vi "Check Device Type.vi"(8 "error in (no error)":errorcluster, 9 "Device Type Name":string, 10 "Device in":refnum<class "Device.lvclass">) -> (0 "error out":errorcluster, 1 "correct Device":bool, 2 "Device out":refnum<class "Device.lvclass">)   [LabVIEW 2011, in "Tinkerforge.lvlib" / "Device.lvclass"]
doc: "This VI is the parent class implementation of \"Check Device Type.vi\"."
uses:
  Device.lvclass
  IP Connection/Type Definitions/Errors.ctl
  IP Connection/IP Connection.lvclass
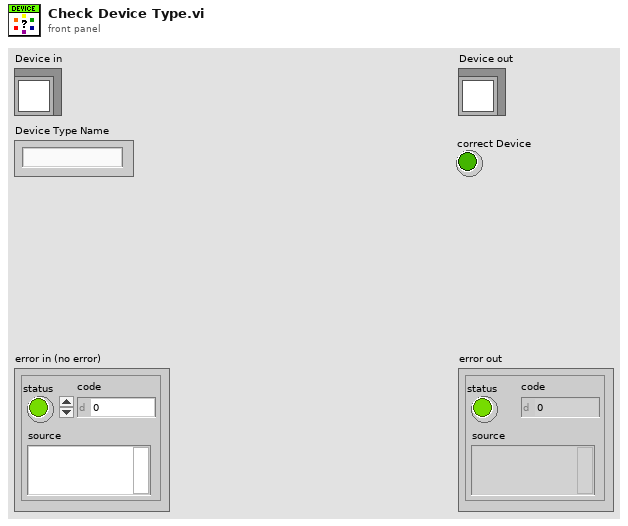
[diagram p1: front panel]
types:
  T1 = typedef "Tinkerforge.lvlib/IP Connection.lvclass/Errors.ctl" = enum16{"Timeout", "Device type incorrect", "Device already added", "Device not existing"}
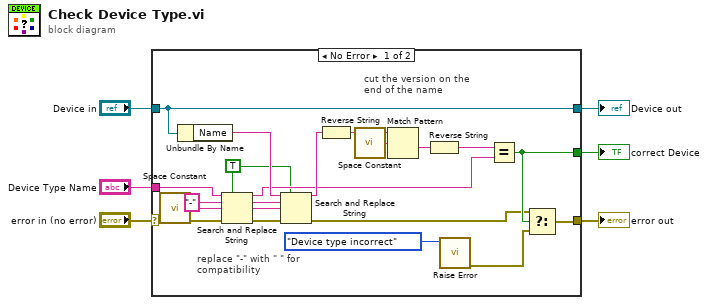
[diagram p0: block diagram]
diagram:
  n1 = case shown="No Error" "error in (no error)" {
    selector: "error in (no error)" -> [w17 w26]
    tunnel: [w18 w26] -> w5
    tunnel: [w24 w25] -> w3
    tunnel: "Device in" -> [w24 w25]
    tunnel: "Device Type Name" -> [w13 _]
    tunnel: [w19 _] -> w1
    frame No Error {
      w9 = TRUE ("replace all? (F)")
      w11 = "-" ("search string")
      # "replace \"-\" with \" \" for\ncompatibility"
      # "cut the version on the\nend of the name"
      n2 = call <vilib>:"Space Constant.vi"() -> ("String"=w10:string)
      n3 = Unbundle By Name(w24) -> ("Name"=w15:string)
      n4 = Search and Replace String(replace all?=w9, input string=w13, search string=w11, replace string=w10) -> (result string=w12:string)  [unwired: 4 in, 3 out]
      n5 = Search and Replace String(replace all?=w9, input string=w15, search string=w11, replace string=w10, error in=w17) -> (result string=w14:string, error out=w16:errorcluster)  [unwired: 3 in, 2 out]
      n6 = Reverse String(1:w14) -> (0:w23:string)
      n7 = call <vilib>:"Space Constant.vi"() -> ("String"=w22:string)
      n8 = Match Pattern(string=w23, regular expression=w22) -> (after substring=w21:string)  [unwired: 1 in, 3 out]
      n9 = Reverse String(1:w21) -> (0:w20:string)
      n10 = call "Raise Error.vi"("Error"=Errors."Device type incorrect") -> ("Error Out"=w7:errorcluster)  [unwired: 10 in]
      n11 = Equal?(x=w20, y=w12) -> (x = y?=w19:bool)
      n12 = Select(t=w16, s=w19, f=w7) -> (s? t:f=w18:errorcluster)
    }
    frame Error {
    }
  }
  "error out" <- w5
  "Device out" <- w3
  "correct Device" <- w1
